vi "Write ConfigDir.vi"(8 "error in (no error)":errorcluster, 10 "ConfigDir":path, 11 "HIJ Vision Camera App In":refnum<class "HIJ Vision Camera App.lvclass">) -> (0 "error out":errorcluster, 3 "HIJ Vision Camera App Out":refnum<class "HIJ Vision Camera App.lvclass">)   [LabVIEW 2020, in "HIJ Vision Camera App.lvlib" / "HIJ Vision Camera App.lvclass"]
uses:
  HIJ Vision Camera App.lvclass
  C:/Users/AlexK/work/LabVIEW Programme/POLARIS CAM Log Abw und E/Submodules/HIJ Vision/Application Base Actors/HIJ Vision Application/HIJ Vision Application/HIJ Vision Application.lvclass
  HIJ Vision Application/HIJ Vision Application/HIJ Vision Application.lvclass/HIJ Vision Application.ctl
  Display Actors/HIJ IMAQdx Display/AF IMAQ Display Messages/Write ConfigDir Msg/Write ConfigDir Msg.lvclass/Write ConfigDir Msg.ctl
  <vilib>/ActorFramework/Message Enqueuer/Message Enqueuer.lvclass/Message Enqueuer.ctl
  HIJ Vision Application/HIJ Vision Application/Read Display Enq.vi
  <vilib>/ActorFramework/Message Enqueuer/Enqueue.vi
  Display Actors/HIJ IMAQdx Display/AF IMAQ Display Messages/Write ConfigDir Msg/Write ConfigDir Msg.lvclass
  C:/Program Files (x86)/National Instruments/LabVIEW 2020/vi.lib/ActorFramework/Message/Message.lvclass
  <vilib>/ActorFramework/Message Priority Queue/Priority Enqueue.vi
  <vilib>/ActorFramework/Message Enqueuer/Message Enqueuer.lvclass
  HIJ Vision Application/HIJ Vision Application/HIJ Vision Application.lvclass
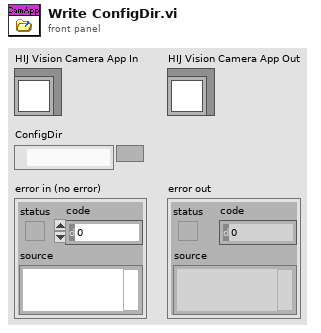
[diagram p1: front panel]
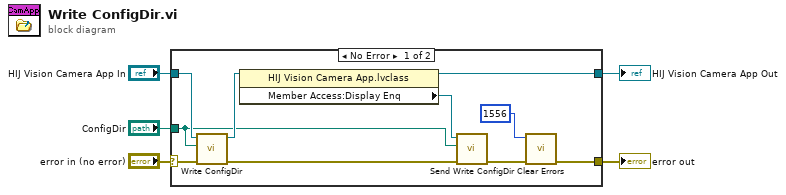
[diagram p0: block diagram]
diagram:
  n1 = case shown="No Error" "error in (no error)" {
    selector: "error in (no error)" -> [w10 w17]
    tunnel: [w7 w17] -> w4
    tunnel: [w14 w16] -> w2
    tunnel: "HIJ Vision Camera App In" -> [w15 w16]
    tunnel: "ConfigDir" -> [w8 _]
    frame No Error {
      n2 = call-parent "Write ConfigDir.vi"("error in (no error)"=w10, "ConfigDir"=w8, "HIJ Vision Application in"=w15) -> ("error out"=w9:errorcluster, "HIJ Vision Application out"=w11:refnum<class "HIJ Vision Camera App.lvclass">)  [unwired: 7 in]
      n3 = property class="HIJ Vision Camera App.lvclass"(reference=w11) -> (reference out=w14:refnum<class "HIJ Vision Camera App.lvclass">, "Member Access:Display Enq"=w13:refnum<class "Message Enqueuer.lvclass">)  [unwired: 1 in, 1 out]
      n4 = call "Send Write ConfigDir.vi"("error in (no error)"=w9, "ConfigDir"=w8, "Message Enqueuer"=w13) -> ("error out"=w12:errorcluster)  [unwired: 7 in, 1 out]
      n5 = call <vilib>:"Clear Errors.vi"("error in (no error)"=w12, "specific error code to clear (0: all)"=1556) -> ("error out"=w7:errorcluster)  [unwired: 4 in, 1 out]
    }
    frame Error {
    }
  }
  "error out" <- w4
  "HIJ Vision Camera App Out" <- w2
